vi "tcp_echo_server.vi"() -> ()   [LabVIEW 2015]
panel:
  in  "Stop Button":bool
  out "incoming message":string
  out "available IP addresses":string[](array[string])
  out "remote port":u16
  out "remote address":string
  # "try tcp listen"
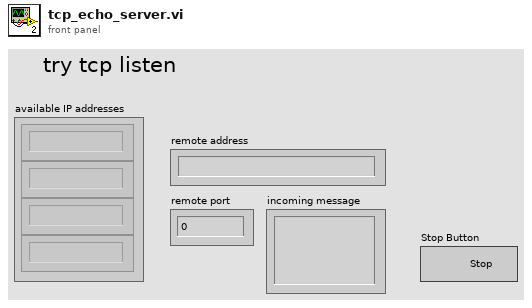
[diagram p1: front panel]
types:
  T1 = enum16{"Standard", "Buffered", "CRLF", "Immediate"}
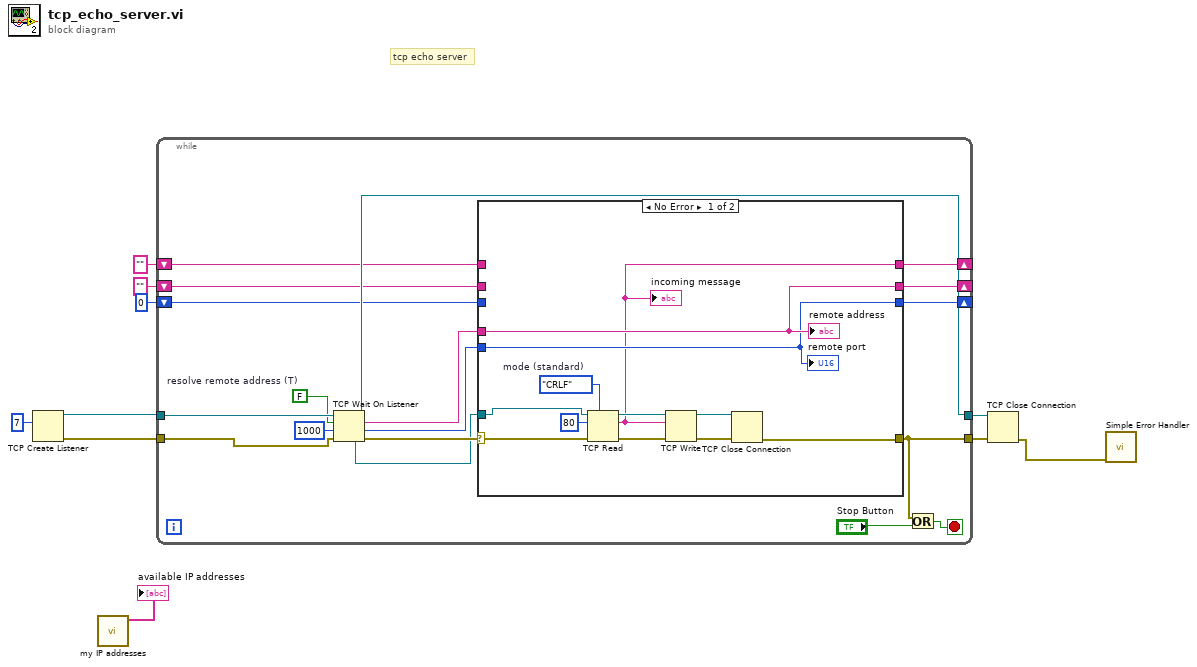
[diagram p0: block diagram]
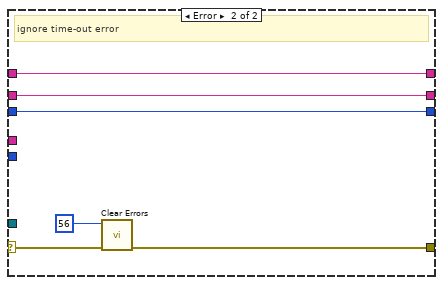
[diagram p2: hidden frame]
diagram:
  # "tcp echo server"
  n1 = TCP Create Listener(10:u16 7 ("port")) -> (0:w9:errorcluster, 3:w8:refnum<k5>)  [unwired: 4 in, 1 out]
  n2 = call "my IP addresses.vi"() -> ("available IP addresses"=→"available IP addresses":string[])  [unwired: 10 in, 1 out]
  n3 = while {
    tunnel: w9 -> [w28]
    tunnel: w8 -> [w27]
    tunnel: [w26] -> w4
    tunnel: [w19] -> w5
    shift-right: [w16] -> _
    shift-left: "" ("remote address") -> [w15]
    shift-right: [w14] -> _
    shift-left: u16 0 ("remote port") -> [w13]
    shift-right: [w12] -> _
    shift-left: "" ("data out") -> [w11]
    stop <- w21 stop-if-true
    w23 = FALSE  # resolve remote address (T)
    n4 = TCP Wait On Listener(8:w28, 9:1000 ("timeout ms (wait forever: -1)"), 10:w23, 11:w27) -> (0:w24:errorcluster, 1:w17:u16, 2:w18:string, 3:w26:refnum<k5>, 4:w22:refnum<k5>)
    n5 = case shown="No Error" w24 {
      selector: w24 -> [w34 w46]
      tunnel: [w35 w44] -> w19
      tunnel: w22 -> [w33 _]
      tunnel: w18 -> [w31 _]
      tunnel: w17 -> [w30 _]
      tunnel: [w31 w43] -> w16
      tunnel: w15 -> [_ w43]
      tunnel: [w30 w42] -> w14
      tunnel: w13 -> [_ w42]
      tunnel: [w29 w41] -> w12
      tunnel: w11 -> [_ w41]
      frame No Error {
        w40 = T1."CRLF"  # mode (standard)
        n6 = TCP Read(connection ID=w33, bytes to read=80, error in (no error)=w34, 7:w40) -> (connection ID out=w37:refnum<k5>, data out=w29:string, error out=w32:errorcluster)  [unwired: 1 in]
        "incoming message" <- w29
        n7 = TCP Write(connection ID=w37, data in=w29, error in (no error)=w32) -> (connection ID out=w36:refnum<k5>, error out=w38:errorcluster)  [unwired: 1 in, 1 out]
        n8 = TCP Close Connection(connection ID=w36, error in (no error)=w38) -> (error out=w35:errorcluster)  [unwired: 1 in, 1 out]
        "remote port" <- w30
        "remote address" <- w31
      }
      frame Error {
        # "ignore time-out error"
        n9 = call <vilib>:"Clear Errors.vi"("error in (no error)"=w46, "specific error code to clear (0: all)"=56) -> ("error out"=w44:errorcluster)  [unwired: 4 in, 1 out]
      }
    }
    n10 = Or(x=w19, y="Stop Button") -> (x .or. y?=w21:bool)
  }
  n11 = TCP Close Connection(connection ID=w4, error in (no error)=w5) -> (error out=w6:errorcluster)  [unwired: 1 in, 1 out]
  n12 = call <vilib>:"Simple Error Handler.vi"("error in (no error)"=w6) -> ()  [unwired: 4 in, 5 out]
